vi "svx_SC Line Facade.vi"(0 "Data In":T9, 2 "Display State In":T4={"X Scale"={"Name"="Horizontal", "format string"="%#.2g", "Major Color"=16777238, "Minor Color"=16777216, "Scale Visible"=TRUE, " Label Visible"=TRUE, "Grid Style"=1, "Maximum"=1.0, "Minimum"=-1.0}, "Y Scale"={"Name"="Vertical", "format string"="%#.2g", "Major Color"=16777238, "Minor Color"=16777216, "Scale Visible"=TRUE, " Label Visible"=TRUE, "Grid Style"=1, "Maximum"=1.0, "Minimum"=-1.0}, "Plot"={"Point Style"=0, "Line Width"=0, "Line Style"=0, "Plot Color"=16860, "Point/fill"=16860}, "Arrow Color"=16860, "Autoscale"=TRUE, "Property Name"=[], "Container Bounds"={"Width"=550, "Height"=313}, "Background color"=16777226, "Annotation List"=[], "Cursor"={"Cursor Point Style"=13, "Cursor Style"=4, "Cursor Line Width"=1, "Cursor Line Style"=0, "Cursor Color"=16711680, "Cursor Name Visible"=TRUE, "Cursor Visible"=TRUE, "Cursor Position"={"X"=0.0, "Y"=0.0}, "Cursor Index"=0, "Lock Cursor Name"=FALSE, "Cursor reference"=0.0}, "size"=0, "Boundary Color"=9868950, "Maximum"=1.0, "Marker Point Style"=2, "Maker Visible"=TRUE, "Marker Color"=16860, "pair strings []"=[], "clearance boundary"=[{"boundary"={"x axis"=0.0, "y axis"=0.0}, "start point"=enum."center"}], "Custom pair name"=FALSE, "selector.visible"=TRUE, "Cursor Release"=refnum, "Children Tags"=[], "open?"=TRUE, "pair index"=[], "Legend Width"=200, " Parents Tags"="", "Label"="", "Legend Background"=16777226, "Legend Font"=16777222, "scale fit"=2, "user strings []"=[], "Item Width"=0, "out of state queue"=refnum, "property nodes"=refnum, "Kind"=enum."X-Scale", "Scale Range Change"=refnum} {"pair index" min=0; "Y Scale"."Minimum" min=0.0; "Y Scale"."Maximum" min=0.0; "X Scale"."Minimum" min=0.0; "X Scale"."Maximum" min=0.0}, 3 "Container State":T8) -> (6 "Data Out":T9, 7 "Display State Out":T4={"X Scale"={"Name"="Horizontal", "format string"="%#.2g", "Major Color"=16777238, "Minor Color"=16777216, "Scale Visible"=TRUE, " Label Visible"=TRUE, "Grid Style"=1, "Maximum"=1.0, "Minimum"=-1.0}, "Y Scale"={"Name"="Vertical", "format string"="%#.2g", "Major Color"=16777238, "Minor Color"=16777216, "Scale Visible"=TRUE, " Label Visible"=TRUE, "Grid Style"=1, "Maximum"=1.0, "Minimum"=-1.0}, "Plot"={"Point Style"=0, "Line Width"=0, "Line Style"=0, "Plot Color"=16860, "Point/fill"=16860}, "Arrow Color"=16860, "Autoscale"=TRUE, "Property Name"=[], "Container Bounds"={"Width"=550, "Height"=313}, "Background color"=16777226, "Annotation List"=[], "Cursor"={"Cursor Point Style"=13, "Cursor Style"=4, "Cursor Line Width"=1, "Cursor Line Style"=0, "Cursor Color"=16711680, "Cursor Name Visible"=TRUE, "Cursor Visible"=TRUE, "Cursor Position"={"X"=0.0, "Y"=0.0}, "Cursor Index"=0, "Lock Cursor Name"=FALSE, "Cursor reference"=0.0}, "size"=0, "Boundary Color"=9868950, "Maximum"=1.0, "Marker Point Style"=2, "Maker Visible"=TRUE, "Marker Color"=16860, "pair strings []"=[], "clearance boundary"=[{"boundary"={"x axis"=0.0, "y axis"=0.0}, "start point"=enum."center"}], "Custom pair name"=FALSE, "selector.visible"=TRUE, "Cursor Release"=refnum, "Children Tags"=[], "open?"=TRUE, "pair index"=[], "Legend Width"=200, " Parents Tags"="", "Label"="", "Legend Background"=16777226, "Legend Font"=16777222, "scale fit"=2, "user strings []"=[], "Item Width"=0, "out of state queue"=refnum, "property nodes"=refnum, "Kind"=enum."X-Scale", "Scale Range Change"=refnum} {"pair index" min=0; "Y Scale"."Minimum" min=0.0; "Y Scale"."Maximum" min=0.0; "X Scale"."Minimum" min=0.0; "X Scale"."Maximum" min=0.0}, 8 "Action":T3)   [LabVIEW 2017, in "SVX SC Line.xctl"]
uses:
  <vilib>/addons/_XControls/Shaft Centerline/SVX SC Line.xctl
  <vilib>/addons/_XControls/Shaft Centerline/subVIs/svx_SC Line Data.ctl
  <vilib>/_xctls/Container State.ctl
  <vilib>/addons/_XControls/Shaft Centerline/subVIs/svx_SC Line State.ctl
  <vilib>/addons/_XControls/Shaft Centerline/subVIs/svx_SC Line Bounds.ctl
  <vilib>/addons/_XControls/Shaft Centerline/subVIs/svx_SC Line Annotation List.ctl
  <vilib>/addons/_XControls/Shaft Centerline/subVIs/svx_SC Line OutState Queue.ctl
  <vilib>/_xctls/Action.ctl
  <vilib>/Utility/miscctls.llb/LVPoint32TypeDef.ctl
  <vilib>/addons/_XControls/Shaft Centerline/subVIs/svx_SC Line Core States.ctl
  <vilib>/Utility/miscctls.llb/LVBoundsTypeDef.ctl
  <vilib>/_xctls/XControlSupport.lvlib
panel:
  out "Coords":T1
  out "cursor info":string
  in  "Tree":string(tree)
  out "Shaft Centerline":T2(graph)
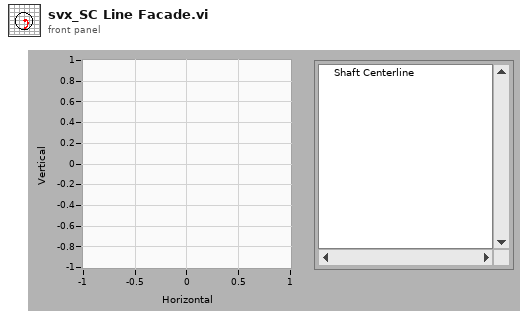
[diagram p1: front panel]
types:
  T1 = typedef "LVPoint32TypeDef.ctl" = cluster{"Horizontal":i32, "Vertical":i32}
  T2 = cluster{"orbit plot X":dbl[], "orbit plot Y":dbl[]}
  T3 = typedef "XControlSupport.lvlib/Action.ctl" = cluster{"Data Changed?":bool, "State Changed?":bool, "Action Name":string}
  T4 = typedef "SVX SC Line.xctl/svx_SC Line State.ctl" = cluster{"X Scale":cluster{"Name":string, "format string":string, "Major Color":u32, "Minor Color":u32, "Scale Visible":bool, " Label Visible":bool, "Grid Style":u16, "Maximum":dbl, "Minimum":dbl}, "Y Scale":cluster{"Name":string, "format string":string, "Major Color":u32, "Minor Color":u32, "Scale Visible":bool, " Label Visible":bool, "Grid Style":u16, "Maximum":dbl, "Minimum":dbl}, "Plot":cluster{"Point Style":u8, "Line Width":u8, "Line Style":u8, "Plot Color":u32, "Point/fill":u32}, "Arrow Color":u32, "Autoscale":bool, "Property Name":string[], "Container Bounds":T5, "Background color":u32, "Annotation List":T6, "Cursor":cluster{"Cursor Point Style":u8, "Cursor Style":u8, "Cursor Line Width":u8, "Cursor Line Style":u8, "Cursor Color":u32, "Cursor Name Visible":bool, "Cursor Visible":bool, "Cursor Position":cluster{"X":dbl, "Y":dbl}, "Cursor Index":i32, "Lock Cursor Name":bool, "Cursor reference":dbl}, "size":i32, "Boundary Color":u32, "Maximum":dbl, "Marker Point Style":u8, "Maker Visible":bool, "Marker Color":u32, "pair strings []":string[], "clearance boundary":cluster{"boundary":cluster{"x axis":dbl, "y axis":dbl}, "start point":enum16{"center", "top", "bottom"}}[], "Custom pair name":bool, "selector.visible":bool, "Cursor Release":refnum<user-event>, "Children Tags":string[], "open?":bool, "pair index":i32[], "Legend Width":u32, " Parents Tags":string, "Label":string, "Legend Background":u32, "Legend Font":u32, "scale fit":u8, "user strings []":string[], "Item Width":u32, "out of state queue":T7, "property nodes":refnum<queue>, "Kind":enum16{"X-Scale", "Y-Scale", "Z-Scale"}, "Scale Range Change":refnum<user-event>}
  T5 = typedef "SVX SC Line.xctl/svx_SC Line Bounds.ctl" = cluster{"Width":u32, "Height":u32}
  T6 = typedef "SVX SC Line.xctl/svx_SC Line Annotation List.ctl" = cluster{"Name":string, "Color":u32, "Style":u8, "Point Style":u8, "Name Visible":bool, "Allow Drag":bool, "Annotation Mode":u32, "Plot":i32, "Index":i32, "Position":cluster{"X":dbl, "Y":dbl}, "X Scale":u32, "Y Scale":u32, "Show Arrow":bool, "Lock Name":bool, "Plot Area":i32, "Label Offset":cluster{"X":dbl, "Y":dbl}}[]
  T7 = typedef "SVX SC Line.xctl/svx_SC Line OutState Queue.ctl" = refnum<queue>
  T8 = typedef "XControlSupport.lvlib/Container State.ctl" = cluster{"Indicator?":bool, "Run Mode?":bool, " Refnum":refnum<vi>}
  T9 = typedef "SVX SC Line.xctl/svx_SC Line Data.ctl" = cluster{"probe x":dbl[], "probe y":dbl[], "reference":dbl[], "attribute":variant}[]
  T10 = cluster{"CursLoc.X":dbl, "Cursloc.Y":dbl, "Cursor.Index":i32, "reference":dbl}
  T11 = typedef "LVBoundsTypeDef.ctl" = cluster{"Width":u32, "Height":u32}
  T12 = typedef "SVX SC Line.xctl/svx_SC Line Core States.ctl" = enum16{"None", "[Axis] Autoscale", "[Image] Update", "[Cursor] Name", "[Plot] Grid&BG", "[Marker] Update", "[Tree] Tags", "[Data] Update", "[Layout] Size", "[Tree] Checkbox", "[Tree] Visible", "[Tree] Open", "[Axis] X", "[Axis] Y", "[Plot] Color", "[Axis] Format String", "[Data] Compare Strings", "[Cursor] Apearance", "[Axis] Name&Visible", "[Tree] Color", "[Data] Index", "[Cursor] Index", "[Axis] Event"}
  T13 = cluster{"boundary":cluster{"x axis":dbl, "y axis":dbl}, "start point":enum16{"center", "top", "bottom"}}[]
  T14 = cluster{"use queue?":bool, "Legend Width":u32, "Cursor reference":dbl, "Cursor Position":cluster{"X":dbl, "Y":dbl}, "pair strings []":string[], "Label":string, "Parents Tags":string, "Children Tags":string[], "Item Width":u32, "Maximum":dbl, "Minimum":dbl, "Maximum":dbl, "Minimum":dbl, "selector.visible":bool, "clearance boundary":cluster{"boundary":cluster{"x axis":dbl, "y axis":dbl}, "start point":enum16{"center", "top", "bottom"}}[], "size":i32}
  T15 = cluster{"probe x":dbl[], "probe y":dbl[], "reference":dbl[], "attribute":variant}
  T16 = typedef "LVRectTypeDef.ctl" = cluster{"Left":i16, "Top":i16, "Right":i16, "Bottom":i16}
  T17 = cluster{"Background color":u32, "actual major":u32, "actual minor":u32, "actual major":u32, "actual minor":u32}
  T18 = cluster{"BG Color":u32, "XScale.MajGrdColor":u32, "XScale.MnrGrdColor":u32, "YScale.MajGrdColor":u32, "YScale.MnrGrdColor":u32}
  T19 = cluster{"Shift":bool, "Ctrl":bool, "Alt":bool, "Cmd":bool, "Opt":bool}
  T20 = cluster{" Refnum":refnum<vi>, "Shaft Centerline":refnum<vi>, "cursor info":refnum<vi>, "Tree":refnum<vi>, "This VI":refnum<vi>}
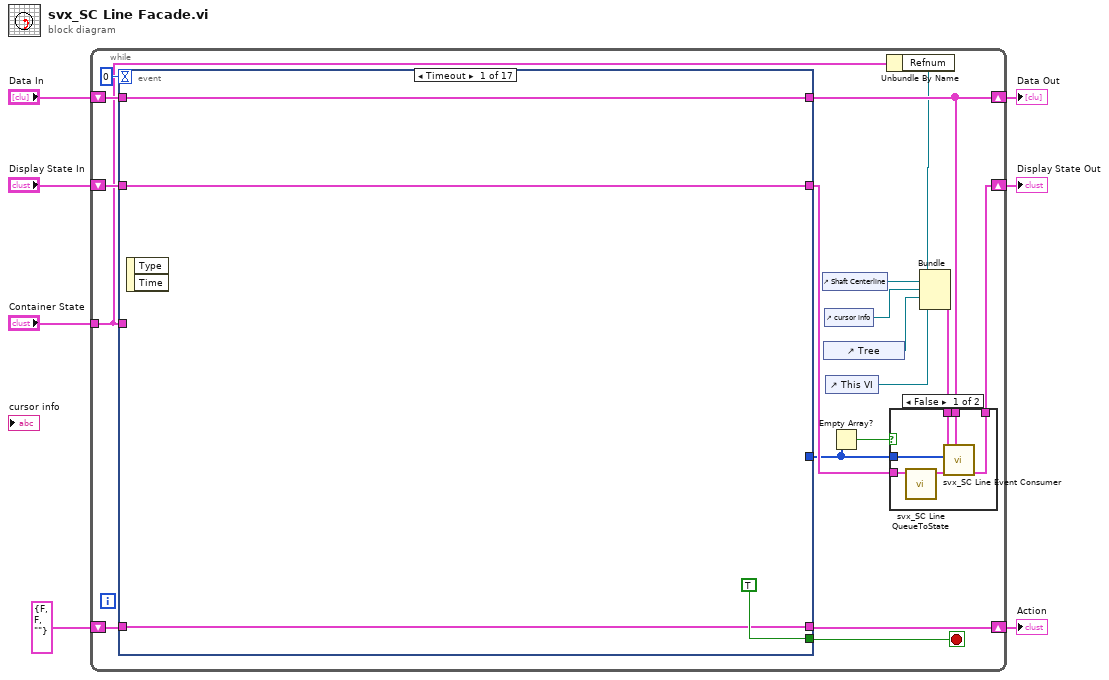
[diagram p0: block diagram]
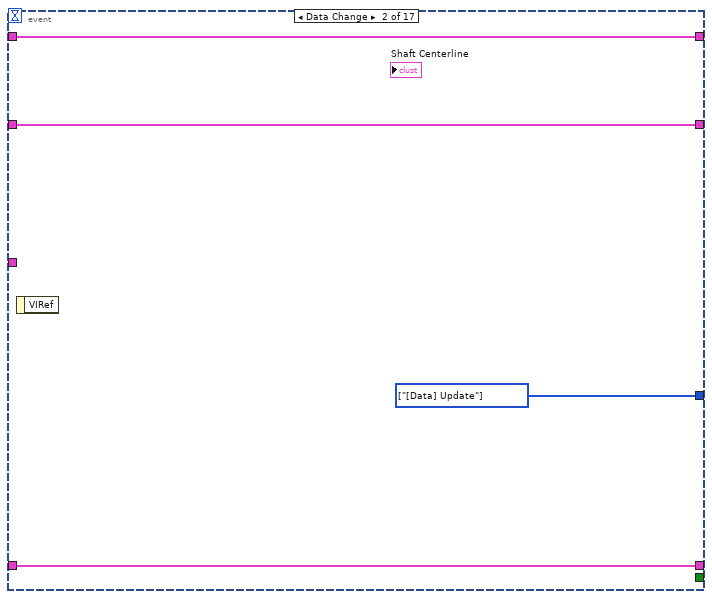
[diagram p3: hidden frame]
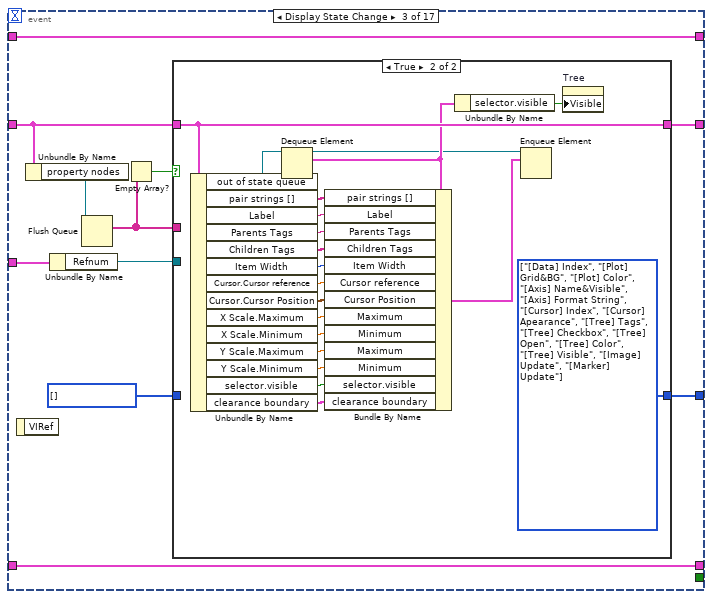
[diagram p4: hidden frame]
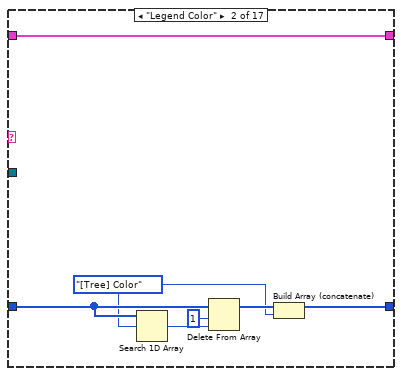
[diagram p6: hidden frame]
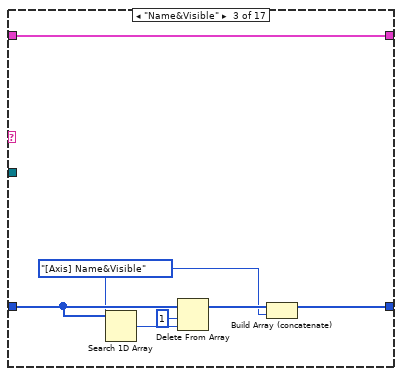
[diagram p7: hidden frame]
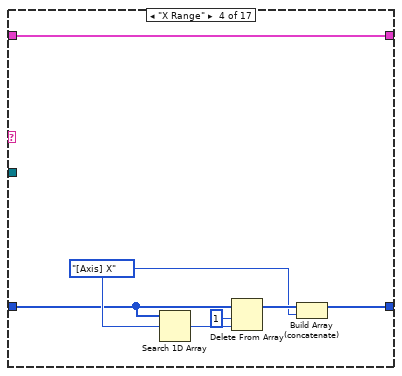
[diagram p8: hidden frame]
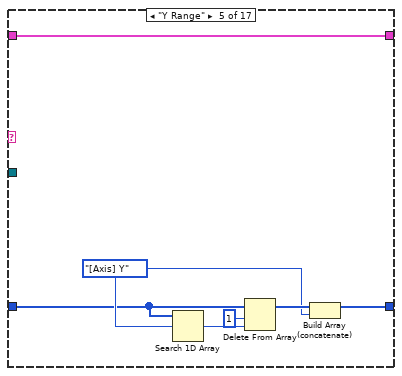
[diagram p9: hidden frame]
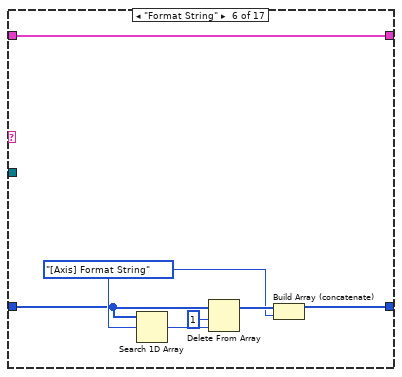
[diagram p10: hidden frame]
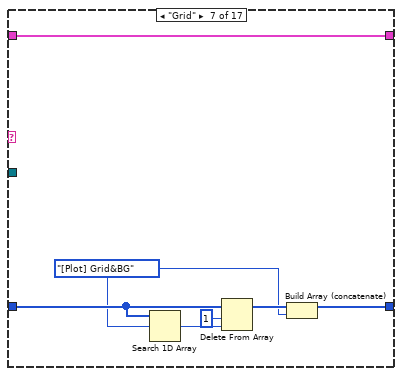
[diagram p11: hidden frame]
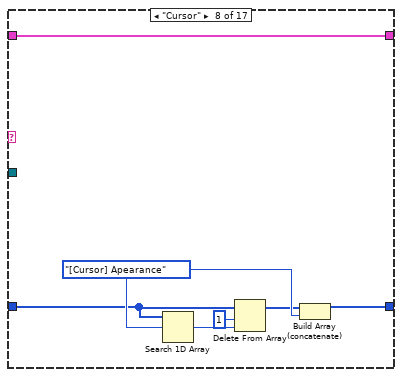
[diagram p12: hidden frame]
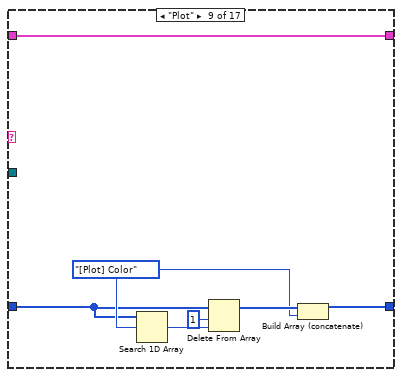
[diagram p13: hidden frame]
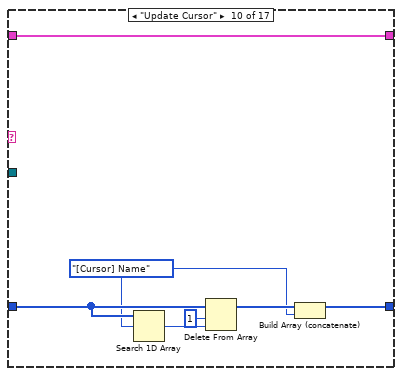
[diagram p14: hidden frame]
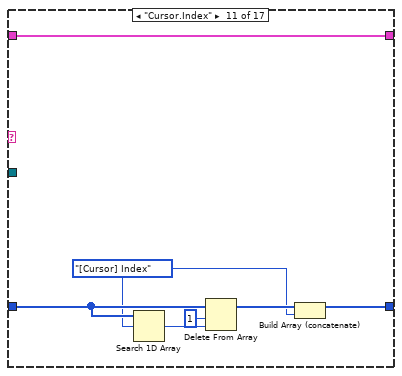
[diagram p15: hidden frame]
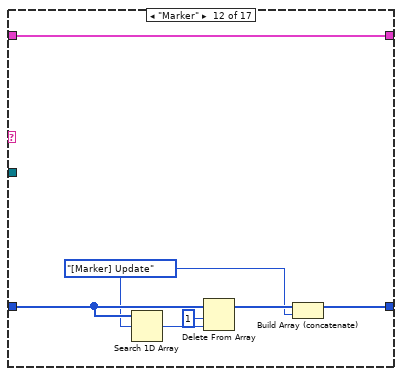
[diagram p16: hidden frame]
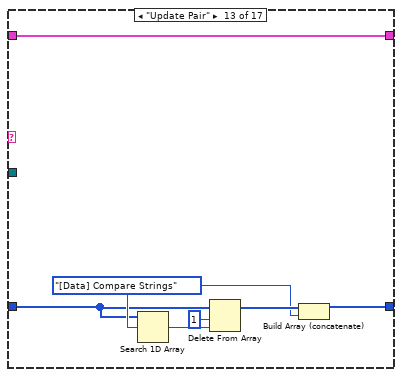
[diagram p17: hidden frame]
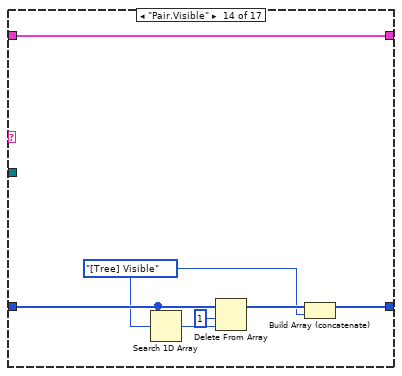
[diagram p18: hidden frame]
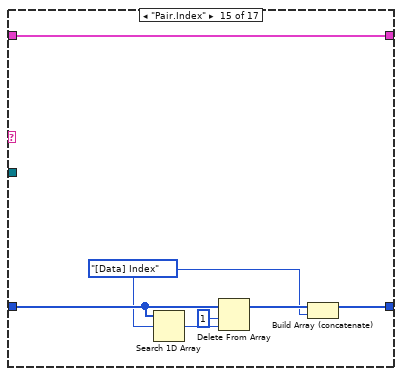
[diagram p19: hidden frame]
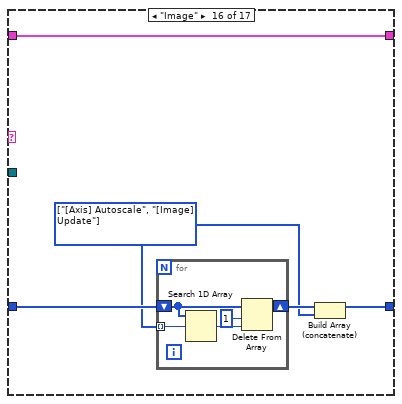
[diagram p20: hidden frame]
diagram:
  n1 = while {
    shift-right: [w17] -> w4
    shift-left: "Display State In" -> [w25]
    tunnel: "Container State" -> [w20]
    shift-right: [w18] -> w7
    shift-left: "Data In" -> [w22]
    shift-right: [w12] -> w2
    shift-left: T3 {"Data Changed?"=FALSE, "State Changed?"=FALSE, "Action Name"=""} ("Action") -> [w21]
    stop <- w24 stop-if-true
    n2 = event shown="[0] Timeout" {
      selector: _ -> [_ _ _ _ _ _ _ _ _ _ _ _ _ _ _ _ _]
      dyn-events: _ -> [_ _ _ _ _ _ _ _ _ _ _ _ _ _ _ _ _]
      timeout: 0 -> [_ _ _ _ _ _ _ _ _ _ _ _ _ _ _ _ _]
      tunnel: w25 -> [w33 w39 w43 w203 w207 w211 w235 w254 w268 w311 w314 w436 w467 w544 w556 w588 w596]
      tunnel: [w33 w39 w48 w203 w207 w209 w235 w254 w267 w311 w321 w435 w466 w541 w550 w588 w596] -> w19
      tunnel: [TRUE _ _ _ _ _ _ _ _ _ _ _ _ _ _ _ _] -> w24
      tunnel: w20 -> [_ _ w50 w204 w208 _ w241 _ _ w309 w319 _ _ _ _ _ _]
      tunnel: w22 -> [w35 w40 w47 w202 w206 w224 w246 w253 w284 w310 w313 w438 w465 w542 w557 w587 w597]
      tunnel: [w35 w40 w47 w202 w206 w224 w246 w253 w284 w310 w313 w437 w465 w542 w557 w587 w597] -> w18
      tunnel: w21 -> [w34 w37 w42 w201 w205 w230 w236 w252 w288 w306 w317 w443 w464 w540 w553 w586 w598]
      tunnel: [_ w38 w49 _ _ w228 w245 _ w269 _ w315 w441 _ _ w551 _ _] -> w11
      tunnel: [w34 w37 w42 w201 w205 w229 w236 w252 w287 w306 w316 w442 w463 w539 w552 w586 w598] -> w12
      event Timeout {
        n3 = event-data() -> ()  [unwired: 1 in, 2 out]
      }
      event Data Change {
        w38 = T12[] [enum."[Data] Update"] items=["None", "[Axis] Autoscale", "[Image] Update", "[Cursor] Name", "[Plot] Grid&BG", "[Marker] Update", "[Tree] Tags", "[Data] Update", "[Layout] Size", "[Tree] Checkbox", "[Tree] Visible", "[Tree] Open", "[Axis] X", "[Axis] Y", "[Plot] Color", "[Axis] Format String", "[Data] Compare Strings", "[Cursor] Apearance", "[Axis] Name&Visible", "[Tree] Color", "[Data] Index", "[Cursor] Index", "[Axis] Event"] ("f")
        n4 = event-data() -> ()  [unwired: 1 in, 1 out]
      }
      event Display State Change {
        w41 = T12[] [] items=["None", "[Axis] Autoscale", "[Image] Update", "[Cursor] Name", "[Plot] Grid&BG", "[Marker] Update", "[Tree] Tags", "[Data] Update", "[Layout] Size", "[Tree] Checkbox", "[Tree] Visible", "[Tree] Open", "[Axis] X", "[Axis] Y", "[Plot] Color", "[Axis] Format String", "[Data] Compare Strings", "[Cursor] Apearance", "[Axis] Name&Visible", "[Tree] Color", "[Data] Index", "[Cursor] Index", "[Axis] Event"]
        n5 = event-data() -> ()  [unwired: 1 in, 1 out]
        n6 = Unbundle By Name(w43) -> ("property nodes"=w45:refnum<queue>)
        n7 = Unbundle By Name(w50) -> ("Refnum"=w46:refnum<vi>)
        n8 = Flush Queue(queue=w45) -> (remaining elements=w44:string[])  [unwired: 1 in, 2 out]
        n9 = Empty Array?(array=w44) -> (empty?=w51:bool)
        n10 = case shown="True" w51 {
          tunnel: w43 -> [w53 w198]
          tunnel: w44 -> [w54 _]
          tunnel: [w57 w200] -> w49
          tunnel: [w56 w198] -> w48
          tunnel: w46 -> [w55 _]
          tunnel: w41 -> [w52 _]
          frame False {
            n11 = for {
              tunnel: w54 -> [w63] mode=indexing
              shift-right: [w61] -> w57
              shift-left: w52 -> [w62]
              shift-right: [w59] -> w56
              shift-left: w53 -> [w60]
              tunnel: w55 -> [w58]
              n12 = case shown="Default" w63 {
                tunnel: w62 -> [w65 w68 w75 w81 w88 w95 w105 w110 w116 w126 w133 w140 w144 w153 w159 w168 w175]
                tunnel: [w65 w67 w74 w80 w87 w94 w104 w108 w115 w125 w132 w139 w143 w152 w157 w167 w174] -> w61
                tunnel: w60 -> [w64 w72 w79 w86 w93 w100 w103 w114 w121 w124 w129 w138 w149 w156 w163 w166 w180]
                tunnel: [w64 w72 w79 w86 w93 w100 w103 w114 w121 w124 w129 w138 w149 w156 w163 w166 w180] -> w59
                tunnel: w58 -> [_ _ _ _ _ _ _ _ _ _ _ _ _ _ _ _ _]
                frame Default {
                }
                frame "Legend Color" {
                  w66 = svx_SC_Line_Core_States."[Tree] Color" ("Property Page User Events")
                  n13 = Search 1D Array(1D array=w68, element=w66) -> (index of element=w71:i32)  [unwired: 1 in]
                  n14 = Delete From Array(array=w68, length=1, index=w71) -> (array with subset deleted=w69:T12[])  [unwired: 1 out]
                  n15 = Build Array (concatenate)(w69, w66) -> (w67:T12[])
                }
                frame "Name&Visible" {
                  w73 = svx_SC_Line_Core_States."[Axis] Name&Visible" ("Property Page User Events")
                  n16 = Search 1D Array(1D array=w75, element=w73) -> (index of element=w78:i32)  [unwired: 1 in]
                  n17 = Delete From Array(array=w75, length=1, index=w78) -> (array with subset deleted=w76:T12[])  [unwired: 1 out]
                  n18 = Build Array (concatenate)(w76, w73) -> (w74:T12[])
                }
                frame "X Range" {
                  w82 = svx_SC_Line_Core_States."[Axis] X" ("Property Page User Events")
                  n19 = Search 1D Array(1D array=w81, element=w82) -> (index of element=w85:i32)  [unwired: 1 in]
                  n20 = Delete From Array(array=w81, length=1, index=w85) -> (array with subset deleted=w83:T12[])  [unwired: 1 out]
                  n21 = Build Array (concatenate)(w83, w82) -> (w80:T12[])
                }
                frame "Y Range" {
                  w89 = svx_SC_Line_Core_States."[Axis] Y" ("Property Page User Events")
                  n22 = Search 1D Array(1D array=w88, element=w89) -> (index of element=w92:i32)  [unwired: 1 in]
                  n23 = Delete From Array(array=w88, length=1, index=w92) -> (array with subset deleted=w90:T12[])  [unwired: 1 out]
                  n24 = Build Array (concatenate)(w90, w89) -> (w87:T12[])
                }
                frame "Format String" {
                  w96 = svx_SC_Line_Core_States."[Axis] Format String" ("Property Page User Events")
                  n25 = Search 1D Array(1D array=w95, element=w96) -> (index of element=w99:i32)  [unwired: 1 in]
                  n26 = Delete From Array(array=w95, length=1, index=w99) -> (array with subset deleted=w97:T12[])  [unwired: 1 out]
                  n27 = Build Array (concatenate)(w97, w96) -> (w94:T12[])
                }
                frame "Grid" {
                  w101 = svx_SC_Line_Core_States."[Plot] Grid&BG" ("Property Page User Events")
                  n28 = Search 1D Array(1D array=w105, element=w101) -> (index of element=w107:i32)  [unwired: 1 in]
                  n29 = Delete From Array(array=w105, length=1, index=w107) -> (array with subset deleted=w102:T12[])  [unwired: 1 out]
                  n30 = Build Array (concatenate)(w102, w101) -> (w104:T12[])
                }
                frame "Cursor" {
                  w111 = svx_SC_Line_Core_States."[Cursor] Apearance" ("Property Page User Events")
                  n31 = Search 1D Array(1D array=w110, element=w111) -> (index of element=w113:i32)  [unwired: 1 in]
                  n32 = Delete From Array(array=w110, length=1, index=w113) -> (array with subset deleted=w109:T12[])  [unwired: 1 out]
                  n33 = Build Array (concatenate)(w109, w111) -> (w108:T12[])
                }
                frame "Plot" {
                  w117 = svx_SC_Line_Core_States."[Plot] Color" ("Property Page User Events")
                  n34 = Search 1D Array(1D array=w116, element=w117) -> (index of element=w120:i32)  [unwired: 1 in]
                  n35 = Delete From Array(array=w116, length=1, index=w120) -> (array with subset deleted=w118:T12[])  [unwired: 1 out]
                  n36 = Build Array (concatenate)(w118, w117) -> (w115:T12[])
                }
                frame "Update Cursor" {
                  w122 = svx_SC_Line_Core_States."[Cursor] Name" ("Property Page User Events")
                  n37 = Search 1D Array(1D array=w126, element=w122) -> (index of element=w128:i32)  [unwired: 1 in]
                  n38 = Delete From Array(array=w126, length=1, index=w128) -> (array with subset deleted=w123:T12[])  [unwired: 1 out]
                  n39 = Build Array (concatenate)(w123, w122) -> (w125:T12[])
                }
                frame "Cursor.Index" {
                  w130 = svx_SC_Line_Core_States."[Cursor] Index" ("Property Page User Events")
                  n40 = Search 1D Array(1D array=w133, element=w130) -> (index of element=w135:i32)  [unwired: 1 in]
                  n41 = Delete From Array(array=w133, length=1, index=w135) -> (array with subset deleted=w131:T12[])  [unwired: 1 out]
                  n42 = Build Array (concatenate)(w131, w130) -> (w132:T12[])
                }
                frame "Marker" {
                  w136 = svx_SC_Line_Core_States."[Marker] Update" ("Property Page User Events")
                  n43 = Search 1D Array(1D array=w140, element=w136) -> (index of element=w142:i32)  [unwired: 1 in]
                  n44 = Delete From Array(array=w140, length=1, index=w142) -> (array with subset deleted=w137:T12[])  [unwired: 1 out]
                  n45 = Build Array (concatenate)(w137, w136) -> (w139:T12[])
                }
                frame "Update Pair" {
                  w145 = svx_SC_Line_Core_States."[Data] Compare Strings" ("Property Page User Events")
                  n46 = Search 1D Array(1D array=w144, element=w145) -> (index of element=w148:i32)  [unwired: 1 in]
                  n47 = Delete From Array(array=w144, length=1, index=w148) -> (array with subset deleted=w146:T12[])  [unwired: 1 out]
                  n48 = Build Array (concatenate)(w146, w145) -> (w143:T12[])
                }
                frame "Pair.Visible" {
                  w150 = svx_SC_Line_Core_States."[Tree] Visible" ("Property Page User Events")
                  n49 = Search 1D Array(1D array=w153, element=w150) -> (index of element=w155:i32)  [unwired: 1 in]
                  n50 = Delete From Array(array=w153, length=1, index=w155) -> (array with subset deleted=w151:T12[])  [unwired: 1 out]
                  n51 = Build Array (concatenate)(w151, w150) -> (w152:T12[])
                }
                frame "Pair.Index" {
                  w158 = svx_SC_Line_Core_States."[Data] Index" ("Property Page User Events")
                  n52 = Search 1D Array(1D array=w159, element=w158) -> (index of element=w162:i32)  [unwired: 1 in]
                  n53 = Delete From Array(array=w159, length=1, index=w162) -> (array with subset deleted=w160:T12[])  [unwired: 1 out]
                  n54 = Build Array (concatenate)(w160, w158) -> (w157:T12[])
                }
                frame "Image" {
                  w164 = T12[] [enum."[Axis] Autoscale", enum."[Image] Update"] items=["None", "[Axis] Autoscale", "[Image] Update", "[Cursor] Name", "[Plot] Grid&BG", "[Marker] Update", "[Tree] Tags", "[Data] Update", "[Layout] Size", "[Tree] Checkbox", "[Tree] Visible", "[Tree] Open", "[Axis] X", "[Axis] Y", "[Plot] Color", "[Axis] Format String", "[Data] Compare Strings", "[Cursor] Apearance", "[Axis] Name&Visible", "[Tree] Color", "[Data] Index", "[Cursor] Index", "[Axis] Event"]
                  n55 = for {
                    shift-right: [w169] -> w165
                    shift-left: w168 -> [w171]
                    tunnel: w164 -> [w170] mode=indexing
                    n56 = Search 1D Array(1D array=w171, element=w170) -> (index of element=w173:i32)  [unwired: 1 in]
                    n57 = Delete From Array(array=w171, length=1, index=w173) -> (array with subset deleted=w169:T12[])  [unwired: 1 out]
                  }
                  n58 = Build Array (concatenate)(w165, w164) -> (w167:T12[])
                }
                frame "Autoscale" {
                  w176 = svx_SC_Line_Core_States."[Axis] Autoscale" ("Property Page User Events")
                  n59 = Search 1D Array(1D array=w175, element=w176) -> (index of element=w179:i32)  [unwired: 1 in]
                  n60 = Delete From Array(array=w175, length=1, index=w179) -> (array with subset deleted=w177:T12[])  [unwired: 1 out]
                  n61 = Build Array (concatenate)(w177, w176) -> (w174:T12[])
                }
              }
            }
          }
          frame True {
            w200 = T12[] [enum."[Data] Index", enum."[Plot] Grid&BG", enum."[Plot] Color", enum."[Axis] Name&Visible", enum."[Axis] Format String", enum."[Cursor] Index", enum."[Cursor] Apearance", enum."[Tree] Tags", enum."[Tree] Checkbox", enum."[Tree] Open", enum."[Tree] Color", enum."[Tree] Visible", enum."[Image] Update", enum."[Marker] Update"] items=["None", "[Axis] Autoscale", "[Image] Update", "[Cursor] Name", "[Plot] Grid&BG", "[Marker] Update", "[Tree] Tags", "[Data] Update", "[Layout] Size", "[Tree] Checkbox", "[Tree] Visible", "[Tree] Open", "[Axis] X", "[Axis] Y", "[Plot] Color", "[Axis] Format String", "[Data] Compare Strings", "[Cursor] Apearance", "[Axis] Name&Visible", "[Tree] Color", "[Data] Index", "[Cursor] Index", "[Axis] Event"]
            n62 = Unbundle By Name(w198) -> ("out of state queue"=w197:T7, "pair strings []"=w195:string[], "Label"=w194:string, "Parents Tags"=w193:string, "Children Tags"=w192:string[], "Item Width"=w191:u32, "Cursor.Cursor reference"=w190:dbl, "Cursor.Cursor Position"=w189:cluster{"X":dbl, "Y":dbl}, "X Scale.Maximum"=w188:dbl, "X Scale.Minimum"=w187:dbl, "Y Scale.Maximum"=w186:dbl, "Y Scale.Minimum"=w185:dbl, "selector.visible"=w184:bool, "clearance boundary"=w183:T13)
            n63 = Dequeue Element(queue=w197) -> (queue out=w182:T7, element=w196:T14)  [unwired: 2 in, 2 out]
            n64 = Bundle By Name(cluster=w196, "pair strings []"=w195, "Label"=w194, "Parents Tags"=w193, "Children Tags"=w192, "Item Width"=w191, "Cursor reference"=w190, "Cursor Position"=w189, "Maximum"=w188, "Minimum"=w187, "Maximum"=w186, "Minimum"=w185, "selector.visible"=w184, "clearance boundary"=w183) -> (w181:T14)
            n65 = Unbundle By Name(w196) -> ("selector.visible"=w199:bool)
            n66 = Enqueue Element(queue=w182, element=w181) -> ()  [unwired: 2 in, 3 out]
            n67 = property on="Tree" class="Tree (strict)"("Visible"=w199) -> ()  [unwired: 2 in, 2 out]
          }
        }
      }
      event Direction Change {
        # "The direction of the XControl changed from a control to an indicator or vice versa. Update the appearance accordingly."
        n68 = event-data() -> ()  [unwired: 1 in, 4 out]
        n69 = Unbundle By Name(w204) -> ()  [unwired: 1 out]
      }
      event Exec State Change {
        # "The VI owning the XControl changed from Edit Mode  to Run Mode or vice versa.\nUpdate the appearance accordingly."
        # "Handle Edit Mode & Run Mode\ncase differently"
        n70 = event-data() -> ()  [unwired: 1 in, 4 out]
        n71 = Unbundle By Name(w208) -> ()  [unwired: 1 out]
      }
      event "Shaft Centerline": Cursor Release {
        w228 = T12[] [enum."[Cursor] Name"] items=["None", "[Axis] Autoscale", "[Image] Update", "[Cursor] Name", "[Plot] Grid&BG", "[Marker] Update", "[Tree] Tags", "[Data] Update", "[Layout] Size", "[Tree] Checkbox", "[Tree] Visible", "[Tree] Open", "[Axis] X", "[Axis] Y", "[Plot] Color", "[Axis] Format String", "[Data] Compare Strings", "[Cursor] Apearance", "[Axis] Name&Visible", "[Tree] Color", "[Data] Index", "[Cursor] Index", "[Axis] Event"] ("f")
        n72 = event-data() -> ("CursLoc"=w219:cluster{"X":dbl, "Y":dbl}, "PointIdx"=w210:i32)  [unwired: 1 in]
        n73 = Unbundle By Name(w211) -> ("out of state queue"=w215:T7, "pair index"=w218:i32[])
        n74 = Index Array(array=w218) -> (element=w217:i32)  [unwired: 1 in]
        n75 = Index Array(array=w224, index=w217) -> (element=w223:T15)
        n76 = Unbundle By Name(w223) -> ("reference"=w222:dbl[])
        n77 = Bundle By Name(cluster=w230, "State Changed?"=TRUE, "Action Name"="Move") -> (w229:T3)
        n78 = Unbundle By Name(w219) -> ("X"=w221:dbl, "Y"=w220:dbl)
        n79 = Index Array(array=w222, index=w210) -> (element=w213:dbl)
        n80 = Dequeue Element(queue=w215) -> (queue out=w216:T7, element=w214:T14)  [unwired: 2 in, 2 out]
        n81 = Bundle By Name(cluster=T10 {"CursLoc.X"=0.0, "Cursloc.Y"=0.0, "Cursor.Index"=0, "reference"=0.0} ("CursLoc"), "CursLoc.X"=w221, "Cursloc.Y"=w220, "Cursor.Index"=w210, "reference"=w213) -> (w226:T10)
        n82 = Bundle By Name(cluster=w214, "Cursor Position"=w219, "Cursor reference"=w213) -> (w212:T14)
        n83 = Bundle By Name(cluster=w211, "Cursor.Cursor Index"=w210) -> (w209:T4)
        n84 = Enqueue Element(queue=w216, element=w212) -> ()  [unwired: 2 in, 3 out]
        n85 = Unbundle By Name(w209) -> ("Cursor Release"=w227:refnum<user-event>)
        n86 = Generate User Event(user event=w227, event data cluster=w226) -> ()  [unwired: 2 in, 2 out]
      }
      event Pane Size {
        w245 = T12[] [enum."[Image] Update", enum."[Marker] Update", enum."[Cursor] Name"] items=["None", "[Axis] Autoscale", "[Image] Update", "[Cursor] Name", "[Plot] Grid&BG", "[Marker] Update", "[Tree] Tags", "[Data] Update", "[Layout] Size", "[Tree] Checkbox", "[Tree] Visible", "[Tree] Open", "[Axis] X", "[Axis] Y", "[Plot] Color", "[Axis] Format String", "[Data] Compare Strings", "[Cursor] Apearance", "[Axis] Name&Visible", "[Tree] Color", "[Data] Index", "[Cursor] Index", "[Axis] Event"] ("f")
        n87 = event-data() -> ("NewBnds.Right"=w250:i16, "NewBnds.Left"=w249:i16, "NewBnds.Bottom"=w248:i16, "NewBnds.Top"=w247:i16)  [unwired: 1 in]
        n88 = Unbundle By Name(w241) -> ("Refnum"=w240:refnum<vi>)
        n89 = control-ref of="Shaft Centerline"() -> (w239:refnum<vi>)
        n90 = control-ref of="Tree"() -> (w237:refnum<vi>)
        n91 = Subtract(x=w250, y=w249) -> (x-y=w244:i16)
        n92 = Subtract(x=w248, y=w247) -> (x-y=w243:i16)
        n93 = Bundle(cluster=T11 {"Width"=0, "Height"=0} ("Plot Area:Size"), "Width"=w244, "Height"=w243) -> (w242:T11)
        n94 = Unbundle By Name(w235) -> ("out of state queue"=w234:T7, "selector.visible"=w238:bool)
        n95 = call <vilib>:"svx_SC Line Resize.vi"("container"=w240, "Bounds"=w242, "Shaft Centerline"=w239, "Tree ref in"=w237, "out of state queue"=w234, "selector.visible"=w238) -> ()  [unwired: 10 in]
      }
      event Shortcut Menu Activation? {
        n96 = event-data() -> ("Coords.Horizontal"=w258:i32, "Coords.Vertical"=w257:i32, "Coords"=w251:T1)  [unwired: 1 in]
        n97 = property on="Shaft Centerline" class="XYGraph (strict)"() -> ("Plot Bounds"=w256:T16)  [unwired: 2 in, 2 out]
        n98 = local write "Coords"(w251) -> ()
        n99 = Unbundle By Name(w256) -> ("Right"=w262:i16, "Left"=w261:i16, "Bottom"=w260:i16, "Top"=w259:i16)
        n100 = In Range and Coerce(upper limit=w262, x=w258, lower limit=w261) -> (In Range?=w265:bool)  [unwired: 1 out]
        n101 = In Range and Coerce(upper limit=w260, x=w257, lower limit=w259) -> (In Range?=w264:bool)  [unwired: 1 out]
        n102 = And(x=w265, y=w264) -> (x .and. y?=w263:bool)
        n103 = Not(x=w263) -> (.not. x?=w255:bool)
        n104 = event-data("Discard?"=w255) -> ()  [unwired: 1 in, 1 out]
      }
      event "Shaft Centerline": Scale Range Change {
        w289 = FALSE ("X Scale.Flipped")
        n105 = event-data() -> ("Kind"=w266:enum16{"X-Scale", "Y-Scale", "Z-Scale"})  [unwired: 1 in]
        n106 = Unbundle By Name(w268) -> ("out of state queue"=w278:T7)
        n107 = Bundle By Name(cluster=w268, "Kind"=w266) -> (w267:T4)
        n108 = property on="Shaft Centerline" class="XYGraph (strict)"("XScale.Flipped"=w289, "YScale.Flipped"=w289) -> ("XScale.Maximum"=w283:dbl, "XScale.Minimum"=w282:dbl, "YScale.Maximum"=w281:dbl, "YScale.Minimum"=w280:dbl)  [unwired: 2 in, 2 out]
        n109 = Dequeue Element(queue=w278) -> (queue out=w279:T7, element=w277:T14)  [unwired: 2 in, 2 out]
        n110 = case shown="\"Y-Scale\"" w266 {
          tunnel: w283 -> [w296 w304]
          tunnel: [w299 w304] -> w273
          tunnel: [w293 w303] -> w276
          tunnel: [w292 w302] -> w275
          tunnel: w281 -> [_ w303]
          tunnel: w280 -> [_ w302]
          tunnel: w282 -> [w298 _]
          tunnel: w277 -> [w294 _]
          tunnel: [svx_SC_Line_Core_States."[Axis] X" ("Property Page User Events") svx_SC_Line_Core_States."[Axis] Y" ("Property Page User Events")] -> w271
          frame "X-Scale", Default {
            n111 = Unbundle By Name(w294) -> ("Maximum"=w293:dbl, "Minimum"=w292:dbl, "Maximum"=w291:dbl)
            n112 = Absolute Value(x=w296) -> (abs(x)=w295:dbl)
            n113 = Absolute Value(x=w298) -> (abs(x)=w297:dbl)
            n114 = Not Equal?(x=w291, y=w295) -> (x != y?=w300:bool)
            n115 = Select(t=w295, s=w300, f=w297) -> (s? t:f=w299:dbl)
          }
          frame "Y-Scale" {
          }
        }
        n116 = Bundle By Name(cluster=w288, "Action Name"="Range Changed", "State Changed?"=TRUE) -> (w287:T3)
        n117 = Negate(x=w273) -> (-x=w272:dbl)
        n118 = Build Array(w271, svx_SC_Line_Core_States."[Axis] Event" ("Property Page User Events")) -> (w269:T12[])
        n119 = Bundle By Name(cluster=w277, "Maximum"=w273, "Minimum"=w272, "Maximum"=w276, "Minimum"=w275) -> (w274:T14)
        n120 = Enqueue Element(queue=w279, element=w274) -> ()  [unwired: 2 in, 3 out]
      }
      event "Shaft Centerline": Shortcut Menu Activation? {
        n121 = event-data() -> ("Coords"=→"Coords":T1, "MenuRef"=w312:refnum<k9>)  [unwired: 1 in]
        n122 = Unbundle By Name(w309) -> ("Refnum"=w308:refnum<vi>, "Run Mode?"=w307:bool)
        n123 = call <vilib>:"svx_SC Line SC Menu.vi"("Run Mode?"=w307, "State"=w311, "Refnum"=w308, "MenuRef"=w312) -> ()  [unwired: 8 in]
        n124 = event-data() -> ()  [unwired: 2 in, 1 out]
      }
      event "Shaft Centerline": Shortcut Menu Selection (User) {
        n125 = event-data() -> ("ItemTag"=w320:string)  [unwired: 1 in]
        n126 = Unbundle By Name(w319) -> ("Refnum"=w318:refnum<vi>)
        n127 = case shown="\"USER_SC_PROPERTIES\"" w320 {
          tunnel: w318 -> [_ w329 w335 _ _ _ _ _ _ _ w412 w422 _]
          tunnel: w317 -> [w323 w325 w331 w344 w353 w362 w371 w380 w392 w401 w406 w421 w434]
          tunnel: w314 -> [w322 w324 w330 w339 w348 w357 w366 w375 w383 w396 w402 w414 w430]
          tunnel: [w322 w324 w330 w338 w347 w356 w365 w374 w383 w395 w403 w423 w428] -> w321
          tunnel: [w323 w325 w331 w343 w352 w361 w370 w379 w391 w400 w405 w420 w433] -> w316
          tunnel: w313 -> [_ _ _ _ _ _ _ _ _ _ w410 w418 _]
          tunnel: [_ _ _ w336 w345 w354 w363 w372 w388 w393 _ _ w427] -> w315
          frame "False", Default {
          }
          frame "USER_SC_LABEL" {
            n128 = property class="Ctl"(reference=w329) -> (reference out=w326:refnum<vi>, "Label.Visible"=w328:bool)  [unwired: 1 in, 1 out]
            n129 = Not(x=w328) -> (.not. x?=w327:bool)
            n130 = property class="Ctl"(reference=w326, "Label.Visible"=w327) -> ()  [unwired: 1 in, 2 out]
          }
          frame "USER_SC_CAPTION" {
            n131 = property class="Ctl"(reference=w335) -> (reference out=w332:refnum<vi>, "Caption.Visible"=w334:bool)  [unwired: 1 in, 1 out]
            n132 = Not(x=w334) -> (.not. x?=w333:bool)
            n133 = property class="Ctl"(reference=w332, "Caption.Visible"=w333) -> ()  [unwired: 1 in, 2 out]
          }
          frame "USER_SC_X_SCALE" {
            w336 = T12[] [enum."[Axis] Name&Visible"] items=["None", "[Axis] Autoscale", "[Image] Update", "[Cursor] Name", "[Plot] Grid&BG", "[Marker] Update", "[Tree] Tags", "[Data] Update", "[Layout] Size", "[Tree] Checkbox", "[Tree] Visible", "[Tree] Open", "[Axis] X", "[Axis] Y", "[Plot] Color", "[Axis] Format String", "[Data] Compare Strings", "[Cursor] Apearance", "[Axis] Name&Visible", "[Tree] Color", "[Data] Index", "[Cursor] Index", "[Axis] Event"] ("f")
            n134 = Unbundle By Name(w339) -> ("X Scale.Scale Visible"=w340:bool)
            n135 = Bundle By Name(cluster=w344, "Action Name"="Show/Hide", "State Changed?"=TRUE) -> (w343:T3)
            n136 = Not(x=w340) -> (.not. x?=w337:bool)
            n137 = Bundle By Name(cluster=w339, "X Scale.Scale Visible"=w337) -> (w338:T4)
          }
          frame "USER_SC_Y_SCALE" {
            w345 = T12[] [enum."[Axis] Name&Visible"] items=["None", "[Axis] Autoscale", "[Image] Update", "[Cursor] Name", "[Plot] Grid&BG", "[Marker] Update", "[Tree] Tags", "[Data] Update", "[Layout] Size", "[Tree] Checkbox", "[Tree] Visible", "[Tree] Open", "[Axis] X", "[Axis] Y", "[Plot] Color", "[Axis] Format String", "[Data] Compare Strings", "[Cursor] Apearance", "[Axis] Name&Visible", "[Tree] Color", "[Data] Index", "[Cursor] Index", "[Axis] Event"] ("f")
            n138 = Unbundle By Name(w348) -> ("Y Scale.Scale Visible"=w349:bool)
            n139 = Bundle By Name(cluster=w353, "Action Name"="Show/Hide", "State Changed?"=TRUE) -> (w352:T3)
            n140 = Not(x=w349) -> (.not. x?=w346:bool)
            n141 = Bundle By Name(cluster=w348, "Y Scale.Scale Visible"=w346) -> (w347:T4)
          }
          frame "USER_SC_CURSOR" {
            w354 = T12[] [enum."[Cursor] Name"] items=["None", "[Axis] Autoscale", "[Image] Update", "[Cursor] Name", "[Plot] Grid&BG", "[Marker] Update", "[Tree] Tags", "[Data] Update", "[Layout] Size", "[Tree] Checkbox", "[Tree] Visible", "[Tree] Open", "[Axis] X", "[Axis] Y", "[Plot] Color", "[Axis] Format String", "[Data] Compare Strings", "[Cursor] Apearance", "[Axis] Name&Visible", "[Tree] Color", "[Data] Index", "[Cursor] Index", "[Axis] Event"] ("f")
            n142 = Unbundle By Name(w357) -> ("Cursor.Cursor Visible"=w358:bool)
            n143 = Bundle By Name(cluster=w362, "Action Name"="Show/Hide", "State Changed?"=TRUE) -> (w361:T3)
            n144 = Not(x=w358) -> (.not. x?=w355:bool)
            n145 = Bundle By Name(cluster=w357, "Cursor.Cursor Visible"=w355) -> (w356:T4)
          }
          frame "USER_SC_CURSORINFO" {
            w363 = T12[] [enum."[Cursor] Name"] items=["None", "[Axis] Autoscale", "[Image] Update", "[Cursor] Name", "[Plot] Grid&BG", "[Marker] Update", "[Tree] Tags", "[Data] Update", "[Layout] Size", "[Tree] Checkbox", "[Tree] Visible", "[Tree] Open", "[Axis] X", "[Axis] Y", "[Plot] Color", "[Axis] Format String", "[Data] Compare Strings", "[Cursor] Apearance", "[Axis] Name&Visible", "[Tree] Color", "[Data] Index", "[Cursor] Index", "[Axis] Event"] ("f")
            n146 = Unbundle By Name(w366) -> ("Cursor.Cursor Name Visible"=w367:bool)
            n147 = Bundle By Name(cluster=w371, "Action Name"="Show/Hide", "State Changed?"=TRUE) -> (w370:T3)
            n148 = Not(x=w367) -> (.not. x?=w364:bool)
            n149 = Bundle By Name(cluster=w366, "Cursor.Cursor Name Visible"=w364) -> (w365:T4)
          }
          frame "USER_SC_LOCK" {
            w372 = T12[] [enum."[Cursor] Name"] items=["None", "[Axis] Autoscale", "[Image] Update", "[Cursor] Name", "[Plot] Grid&BG", "[Marker] Update", "[Tree] Tags", "[Data] Update", "[Layout] Size", "[Tree] Checkbox", "[Tree] Visible", "[Tree] Open", "[Axis] X", "[Axis] Y", "[Plot] Color", "[Axis] Format String", "[Data] Compare Strings", "[Cursor] Apearance", "[Axis] Name&Visible", "[Tree] Color", "[Data] Index", "[Cursor] Index", "[Axis] Event"] ("f")
            n150 = Unbundle By Name(w375) -> ("Cursor.Lock Cursor Name"=w376:bool)
            n151 = Bundle By Name(cluster=w380, "Action Name"="Lock Cursor", "State Changed?"=TRUE) -> (w379:T3)
            n152 = Not(x=w376) -> (.not. x?=w373:bool)
            n153 = Bundle By Name(cluster=w375, "Cursor.Lock Cursor Name"=w373) -> (w374:T4)
          }
          frame "USER_SC_SELECTOR" {
            w388 = T12[] [enum."[Tree] Visible"] items=["None", "[Axis] Autoscale", "[Image] Update", "[Cursor] Name", "[Plot] Grid&BG", "[Marker] Update", "[Tree] Tags", "[Data] Update", "[Layout] Size", "[Tree] Checkbox", "[Tree] Visible", "[Tree] Open", "[Axis] X", "[Axis] Y", "[Plot] Color", "[Axis] Format String", "[Data] Compare Strings", "[Cursor] Apearance", "[Axis] Name&Visible", "[Tree] Color", "[Data] Index", "[Cursor] Index", "[Axis] Event"] ("f")
            n154 = Unbundle By Name(w383) -> ("out of state queue"=w385:T7)
            n155 = Bundle By Name(cluster=w392, "Action Name"="Show Selector", "State Changed?"=TRUE) -> (w391:T3)
            n156 = Dequeue Element(queue=w385) -> (queue out=w384:T7, element=w381:T14)  [unwired: 2 in, 2 out]
            n157 = Unbundle By Name(w381) -> ("selector.visible"=w386:bool)
            n158 = Not(x=w386) -> (.not. x?=w387:bool)
            n159 = Bundle By Name(cluster=w381, "selector.visible"=w387) -> (w382:T14)
            n160 = Enqueue Element(queue=w384, element=w382) -> ()  [unwired: 2 in, 3 out]
          }
          frame "USER_SC_MARKER" {
            w393 = T12[] [enum."[Marker] Update"] items=["None", "[Axis] Autoscale", "[Image] Update", "[Cursor] Name", "[Plot] Grid&BG", "[Marker] Update", "[Tree] Tags", "[Data] Update", "[Layout] Size", "[Tree] Checkbox", "[Tree] Visible", "[Tree] Open", "[Axis] X", "[Axis] Y", "[Plot] Color", "[Axis] Format String", "[Data] Compare Strings", "[Cursor] Apearance", "[Axis] Name&Visible", "[Tree] Color", "[Data] Index", "[Cursor] Index", "[Axis] Event"] ("f")
            n161 = Unbundle By Name(w396) -> ("Maker Visible"=w397:bool)
            n162 = Bundle By Name(cluster=w401, "Action Name"="Show/Hide", "State Changed?"=TRUE) -> (w400:T3)
            n163 = Not(x=w397) -> (.not. x?=w394:bool)
            n164 = Bundle By Name(cluster=w396, "Maker Visible"=w394) -> (w395:T4)
          }
          frame "USER_SC_PROPERTIES" {
            n165 = control-ref of="Shaft Centerline"() -> (w411:refnum<vi>)
            n166 = control-ref of="Tree"() -> (w408:refnum<vi>)
            n167 = control-ref of="cursor info"() -> (w409:refnum<vi>)
            n168 = call <vilib>:"svx_SC Line QueueToState.vi"("State in"=w402) -> ("State out"=w404:T4)  [unwired: 10 in]
            n169 = call <vilib>:"svx_SC Line Property Dialog.vi"("Refnum"=w412, "State In"=w404, "Clearance Only?"=FALSE, "SC Line in"=w411, "cursor info"=w409, "Tree"=w408, "Data"=w410, "Action in"=w406) -> ("State Out"=w403:T4, "Action out"=w405:T3)  [unwired: 6 in]
          }
          frame "USER_SC_CB" {
            n170 = control-ref of="Shaft Centerline"() -> (w419:refnum<vi>)
            n171 = control-ref of="Tree"() -> (w416:refnum<vi>)
            n172 = control-ref of="cursor info"() -> (w417:refnum<vi>)
            n173 = call <vilib>:"svx_SC Line QueueToState.vi"("State in"=w414) -> ("State out"=w413:T4)  [unwired: 10 in]
            n174 = call <vilib>:"svx_SC Line Property Dialog.vi"("Refnum"=w422, "State In"=w413, "Clearance Only?"=TRUE, "SC Line in"=w419, "cursor info"=w417, "Tree"=w416, "Data"=w418, "Action in"=w421) -> ("State Out"=w423:T4, "Action out"=w420:T3)  [unwired: 6 in]
          }
          frame "USER_SC_AUTOSCALE" {
            w427 = T12[] [enum."[Axis] Autoscale"] items=["None", "[Axis] Autoscale", "[Image] Update", "[Cursor] Name", "[Plot] Grid&BG", "[Marker] Update", "[Tree] Tags", "[Data] Update", "[Layout] Size", "[Tree] Checkbox", "[Tree] Visible", "[Tree] Open", "[Axis] X", "[Axis] Y", "[Plot] Color", "[Axis] Format String", "[Data] Compare Strings", "[Cursor] Apearance", "[Axis] Name&Visible", "[Tree] Color", "[Data] Index", "[Cursor] Index", "[Axis] Event"] ("f")
            n175 = Unbundle By Name(w430) -> ("Autoscale"=w431:bool)
            n176 = Bundle By Name(cluster=w434, "Action Name"="Graph Scale Option", "State Changed?"=TRUE) -> (w433:T3)
            n177 = Not(x=w431) -> (.not. x?=w426:bool)
            n178 = Boolean To (0,1)(Boolean=w426) -> (0, 1=w425:i16)
            n179 = Add(x=w425, y=w425) -> (x+y=w424:i16)
            n180 = Bundle By Name(cluster=w430, "Autoscale"=w426, "scale fit"=w424) -> (w428:T4)
          }
        }
      }
      event "Shaft Centerline": Shortcut Menu Selection? (App) {
        n181 = event-data() -> ("ItemTag"=w440:string)  [unwired: 1 in]
        n182 = case shown="\"APP_SC_CLEAR_GRAPH\"" w440 {
          tunnel: w443 -> [w446 w459]
          tunnel: [w446 w458] -> w442
          tunnel: w438 -> [w445 _]
          tunnel: [_ w456] -> w441
          tunnel: [_ TRUE ("Discard?")] -> w439
          tunnel: [w445 T9 [] ("Data In")] -> w437
          tunnel: w436 -> [w444 w447]
          tunnel: [w444 w447] -> w435
          frame Default {
          }
          frame "APP_SC_CLEAR_GRAPH" {
            w456 = T12[] [enum."[Data] Update", enum."[Image] Update"] items=["None", "[Axis] Autoscale", "[Image] Update", "[Cursor] Name", "[Plot] Grid&BG", "[Marker] Update", "[Tree] Tags", "[Data] Update", "[Layout] Size", "[Tree] Checkbox", "[Tree] Visible", "[Tree] Open", "[Axis] X", "[Axis] Y", "[Plot] Color", "[Axis] Format String", "[Data] Compare Strings", "[Cursor] Apearance", "[Axis] Name&Visible", "[Tree] Color", "[Data] Index", "[Cursor] Index", "[Axis] Event"] ("f")
            w453 = TRUE ("State Changed?")
            n183 = Unbundle By Name(w447) -> ("out of state queue"=w449:T7)
            n184 = Dequeue Element(queue=w449) -> (queue out=w451:T7, element=w452:T14)  [unwired: 2 in, 2 out]
            n185 = Bundle By Name(cluster=w459, "Action Name"="Clear Graph", "Data Changed?"=w453, "State Changed?"=w453) -> (w458:T3)
            n186 = Bundle By Name(cluster=w452, "clearance boundary"=T13 []) -> (w450:T14)
            n187 = Enqueue Element(queue=w451, element=w450) -> ()  [unwired: 2 in, 3 out]
          }
        }
        n188 = event-data("Discard?"=w439) -> ()  [unwired: 1 in, 1 out]
      }
      event "Shaft Centerline": Mouse Down {
        n189 = event-data() -> ("Button"=w461:u16)  [unwired: 1 in]
        n190 = Equal?(x=u16 1, y=w461) -> (x = y?=w460:bool)
        n191 = case shown="True" w460 {
          tunnel: w467 -> [w469 w498]
          tunnel: [w469 w497] -> w466
          tunnel: [w468 w495] -> w463
          tunnel: w464 -> [w468 w496]
          frame False {
          }
          frame True {
            n192 = Unbundle By Name(w498) -> ("Background color"=w494:u32, "X Scale.Grid Style"=w486:u16, "X Scale.Major Color"=w485:u32, "X Scale.Minor Color"=w484:u32, "Y Scale.Grid Style"=w480:u16, "Y Scale.Major Color"=w477:u32, "Y Scale.Minor Color"=w476:u32)
            n193 = property on="Shaft Centerline" class="XYGraph (strict)"() -> ("BG Color"=w493:u32, "XScale.MajGrdColor"=w491:u32, "XScale.MnrGrdColor"=w490:u32, "YScale.MajGrdColor"=w489:u32, "YScale.MnrGrdColor"=w488:u32)  [unwired: 2 in, 2 out]
            n194 = call <vilib>:"svx_SC Line Manage Grid.vi"("Minor Color"=w484, "enable update?"=FALSE, "Major Color"=w485, "Axis"=enum16{"X-Scale", "Y-Scale", "Z-Scale"}."X-Scale", "Grid Style"=w486) -> ("actual minor"=w481:u32, "actual major"=w482:u32)  [unwired: 4 in, 1 out]
            n195 = call <vilib>:"svx_SC Line Manage Grid.vi"("Minor Color"=w476, "enable update?"=FALSE, "Major Color"=w477, "Axis"=enum16{"X-Scale", "Y-Scale", "Z-Scale"}."Y-Scale", "Grid Style"=w480) -> ("actual minor"=w474:u32, "actual major"=w475:u32)  [unwired: 4 in, 1 out]
            n196 = Bundle("Background color"=w494, "actual major"=w482, "actual minor"=w481, "actual major"=w475, "actual minor"=w474) -> (w473:T17)  [unwired: 1 in]
            n197 = Bundle("BG Color"=w493, "XScale.MajGrdColor"=w491, "XScale.MnrGrdColor"=w490, "YScale.MajGrdColor"=w489, "YScale.MnrGrdColor"=w488) -> (w492:T18)  [unwired: 1 in]
            n198 = Not Equal?(x=w473, y=w492) -> (x != y?=w470:cluster{bool, bool, bool, bool, bool})
            n199 = Cluster To Array(cluster=w470) -> (array=w472:bool[])
            n200 = Or Array Elements(Boolean array=w472) -> (logical OR=w471:bool)
            n201 = case shown="True" w471 {
              tunnel: w498 -> [w500 w516]
              tunnel: [w500 w515] -> w497
              tunnel: w496 -> [w499 w514]
              tunnel: [w499 w513] -> w495
              tunnel: w493 -> [_ w510]
              tunnel: w491 -> [_ w509]
              tunnel: w490 -> [_ w508]
              tunnel: w489 -> [_ w507]
              tunnel: w488 -> [_ w506]
              tunnel: w470 -> [_ w505]
              frame False {
              }
              frame True {
                n202 = Unbundle(w505) -> (w504:bool, w503:bool, w502:bool)  [unwired: 2 out]
                n203 = Or(x=w503, y=w502) -> (x .or. y?=w501:bool)
                n204 = case shown="False" w504 {
                  tunnel: w516 -> [w519 w526]
                  tunnel: [w518 w525] -> w515
                  tunnel: w510 -> [w517 _]
                  tunnel: w509 -> [_ w520]
                  tunnel: w508 -> [_ w524]
                  tunnel: w507 -> [_ w523]
                  tunnel: w506 -> [_ w522]
                  tunnel: w501 -> [_ w521]
                  frame True {
                    n205 = Bundle By Name(cluster=w519, "Background color"=w517) -> (w518:T4)
                  }
                  frame False {
                    n206 = case shown="False" w521 {
                      tunnel: w526 -> [w531 w536]
                      tunnel: [w529 w535] -> w525
                      tunnel: w524 -> [_ w534]
                      tunnel: w523 -> [w530 _]
                      tunnel: w522 -> [w528 _]
                      tunnel: w520 -> [_ w533]
                      frame False {
                        n207 = Bundle By Name(cluster=w531, "Y Scale.Grid Style"=u16 2, "Y Scale.Major Color"=w530, "Y Scale.Minor Color"=w528) -> (w529:T4)
                      }
                      frame True {
                        n208 = Bundle By Name(cluster=w536, "X Scale.Grid Style"=u16 2, "X Scale.Major Color"=w533, "X Scale.Minor Color"=w534) -> (w535:T4)
                      }
                    }
                  }
                }
                n209 = Bundle By Name(cluster=w514, "State Changed?"=TRUE, "Action Name"="Color Changed") -> (w513:T3)
              }
            }
          }
        }
      }
      event "Tree": event #0x1e; "Tree": Item Close {
        n210 = event-data() -> ("Tag"=w545:string)  [unwired: 1 in]
        n211 = property on="Tree" class="Tree (strict)"("Active Item Tag"=w545) -> ("Open?"=w543:bool)  [unwired: 2 in, 2 out]
        n212 = Bundle By Name(cluster=w540, "State Changed?"=TRUE, "Action Name"="Item Open") -> (w539:T3)
        n213 = Bundle By Name(cluster=w544, "open?"=w543) -> (w541:T4)
      }
      event "Tree": Mouse Down {
        n214 = event-data() -> ("CtlRef"=w559:refnum<vi>, "Coords"=w558:T1)  [unwired: 1 in]
        n215 = Unbundle By Name(w556) -> ("out of state queue"=w548:T7, "Legend Background"=w549:u32)
        n216 = Preview Queue Element(queue=w548) -> (element=w547:T14)  [unwired: 2 in, 3 out]
        n217 = Unbundle By Name(w547) -> ("Children Tags"=w546:string[])
        n218 = call <vilib>:"svx_SC Line CheckboxToIndex.vi"("All Children Tags"=w546, "Coords"=w558, "Tree ref in"=w559) -> ("State Changed?"=w554:bool, "index"=w555:i32[])  [unwired: 6 in, 1 out]
        n219 = case shown="True" w554 {
          tunnel: w556 -> [w564 w584]
          tunnel: w555 -> [_ w583]
          tunnel: [w563 w582] -> w550
          tunnel: w553 -> [w561 w581]
          tunnel: [w562 w580] -> w552
          tunnel: [_ w579] -> w551
          tunnel: w549 -> [w566 _]
          frame False {
            w567 = -2 ("Active Cell:Active Column Number")
            n220 = property on="Tree" class="Tree (strict)"("ActiveColNum"=w567, "Active Item Row Number"=w567) -> ("CellBG"=w560:u32)  [unwired: 2 in, 2 out]
            n221 = Equal?(x=w560, y=w566) -> (x = y?=w565:bool)
            n222 = case shown="False" w565 {
              tunnel: w564 -> [w570 w576]
              tunnel: [w568 w576] -> w563
              tunnel: [w571 w575] -> w562
              tunnel: w561 -> [w572 w575]
              tunnel: w560 -> [w569 _]
              frame False {
                n223 = Bundle By Name(cluster=w572, "State Changed?"=TRUE, "Action Name"="Color Change") -> (w571:T3)
                n224 = Bundle By Name(cluster=w570, "Legend Background"=w569) -> (w568:T4)
              }
              frame True {
              }
            }
          }
          frame True {
            w579 = T12[] [enum."[Data] Index"] items=["None", "[Axis] Autoscale", "[Image] Update", "[Cursor] Name", "[Plot] Grid&BG", "[Marker] Update", "[Tree] Tags", "[Data] Update", "[Layout] Size", "[Tree] Checkbox", "[Tree] Visible", "[Tree] Open", "[Axis] X", "[Axis] Y", "[Plot] Color", "[Axis] Format String", "[Data] Compare Strings", "[Cursor] Apearance", "[Axis] Name&Visible", "[Tree] Color", "[Data] Index", "[Cursor] Index", "[Axis] Event"] ("array")
            n225 = Bundle By Name(cluster=w584, "pair index"=w583) -> (w582:T4)
            n226 = Bundle By Name(cluster=w581, "State Changed?"=TRUE, "Action Name"="Index Changed") -> (w580:T3)
          }
        }
      }
      event "Tree", "cursor info": Shortcut Menu Activation? {
        n227 = event-data() -> ("Coords"=w585:T1)  [unwired: 1 in]
        n228 = local write "Coords"(w585) -> ()
        n229 = event-data("Discard?"=TRUE) -> ()  [unwired: 1 in, 1 out]
      }
      event Mouse Down? {
        n230 = event-data() -> ("Button"=w592:u16, "Mods"=w595:cluster{"Double Click":bool, "Menu Key":bool}, "PlatMods"=w593:T19, "Coords"=w590:T1)  [unwired: 1 in]
        n231 = case shown="1" w592 {
          tunnel: w595 -> [w603 w607]
          tunnel: [w606 w607] -> w594
          tunnel: w590 -> [w604 _]
          frame 1 {
            n232 = local read "Coords"() -> (w605:T1)
            n233 = Unbundle By Name(w603) -> ("Double Click"=w600:bool)
            n234 = Equal?(x=w604, y=w605) -> (x = y?=w601:bool)
            n235 = Select(t=FALSE ("Double Click"), s=w601, f=w600) -> (s? t:f=w599:bool)
            n236 = Bundle By Name(cluster=w603, "Double Click"=w599) -> (w606:cluster{"Double Click":bool, "Menu Key":bool})
          }
          frame 0, Default {
          }
        }
        n237 = event-data("Button"=w592, "Mods"=w594, "PlatMods"=w593, "Discard?"=FALSE) -> ()  [unwired: 1 in, 1 out]
      }
    }
    n238 = control-ref of="Shaft Centerline"() -> (w15:refnum<vi>)
    n239 = control-ref of="Tree"() -> (w9:refnum<vi>)
    n240 = control-ref of="cursor info"() -> (w16:refnum<vi>)
    n241 = control-ref of="This VI"() -> (w14:refnum<vi>)
    n242 = Empty Array?(array=w11) -> (empty?=w10:bool)
    n243 = Unbundle By Name(w20) -> ("Refnum"=w8:refnum<vi>)
    n244 = Bundle("Refnum"=w8, "Shaft Centerline"=w15, "cursor info"=w16, "Tree"=w9, "This VI"=w14) -> (w13:T20)  [unwired: 1 in]
    n245 = case shown="False" w10 {
      tunnel: w19 -> [w27 w32]
      tunnel: w18 -> [w31 _]
      tunnel: [w30 w32] -> w17
      tunnel: w13 -> [w29 _]
      tunnel: w11 -> [w28 _]
      frame False {
        n246 = call <vilib>:"svx_SC Line QueueToState.vi"("State in"=w27) -> ("State out"=w26:T4)  [unwired: 10 in]
        n247 = call <vilib>:"svx_SC Line Event Consumer.vi"("shaft centerline"=w31, "State in"=w26, "events"=w28, "references"=w29) -> ("State out"=w30:T4)  [unwired: 7 in]
      }
      frame True {
      }
    }
  }
  "Display State Out" <- w4
  "Data Out" <- w7
  "Action" <- w2
